vi "LSMcontroller_v59_PIzstage.vi"() -> ()   [LabVIEW 2015] (continued)
                                tunnel: w2761 -> [w2765 w2785]
                                tunnel: w2762 -> [_ w2791]
                                frame False {
                                w2769 = u16 0 items=["unsigned binary", "offset binary", "2's complement"] ("data format (offset binary)")
                                n482 = Initialize Array(sgl 0.0, w2765) -> (w2772:sgl[])
                                n483 = Replace Array Subset(array=w2772, new element=sgl 1.0, index=0) -> (w2770:sgl[])
                                n484 = Reciprocal(x=w2775) -> (1/x=w2776:sgl)
                                n485 = Bundle By Name("Y"=w2770, "dt"=w2776) -> (w2767:waveform(sgl))  [unwired: 1 in]
                                n486 = call-poly <vilib>:"Analog to Digital.vi"("data format (offset binary)"=w2769, "compress digital (T)"=TRUE, "full-scale range (pk-pk)"=1.0, "resolution (16 bit)"=1, "analog waveform"=w2767) -> ("digital waveform"=w2766:digitalwaveform)  [unwired: 3 in, 3 out]
                                }
                                frame True {
                                w2782 = u16 0 items=["unsigned binary", "offset binary", "2's complement"] ("data format (offset binary)")
                                n487 = To Double Precision Float(number=w2785) -> (double precision float=w2792:dbl)
                                n488 = Initialize Array(sgl 0.0, w2785) -> (w2787:sgl[])
                                n489 = Divide(x=w2791, y=w2792) -> (x/y=w2789:dbl)
                                n490 = Round Toward +Infinity(x=w2789) -> (ceil(x): smallest int >= x=w2790:dbl)
                                n491 = Replace Array Subset(array=w2787, new element=sgl 1.0, index=0) -> (w2784:sgl[])
                                n492 = for {
                                N: w2790 -> [_]
                                tunnel: w2784 -> [w2796]
                                tunnel: [w2796] -> w2793 mode=concatenating
                                }
                                n493 = Reciprocal(x=w2794) -> (1/x=w2795:sgl)
                                n494 = Bundle By Name("Y"=w2793, "dt"=w2795) -> (w2780:waveform(sgl))  [unwired: 1 in]
                                n495 = call-poly <vilib>:"Analog to Digital.vi"("data format (offset binary)"=w2782, "compress digital (T)"=TRUE, "full-scale range (pk-pk)"=1.0, "resolution (16 bit)"=1, "analog waveform"=w2780) -> ("digital waveform"=w2779:digitalwaveform)  [unwired: 3 in, 3 out]
                                }
                                }
                                n496 = Build Array (concatenate)(w2754, w2756) -> (w2752:digitalwaveform[])
                                n497 = call "waveformsDObuffer.vi"("DO wf in"=w2752, "command"="set") -> ()  [unwired: 1 out]
                                }
                                frame 2 {
                                n498 = call "waveformsDObuffer.vi"("command"="get") -> ("DO wf out"=w2800:digitalwaveform[])  [unwired: 1 in]
                                n499 = Delete From Array(array=w2800, length=1, index=w2803) -> (deleted portion=w2798:digitalwaveform[], array with subset deleted=w2797:digitalwaveform[])
                                n500 = call "waveformsDObuffer.vi"("DO wf in"=w2797, "command"="set") -> ()  [unwired: 1 out]
                                }
                                frame 3, Default {
                                }
                                frame 0 {
                                n501 = local read "Measurement"() -> (w2806:T4)
                                n502 = To Unsigned Long Integer(number=w2806) -> (unsigned 32bit integer=w2805:u32)
                                n503 = case shown="5..7" w2805 {
                                tunnel: w2807 -> [_ w2810]
                                tunnel: [_ w2809] -> w2804
                                frame 0..4, Default {
                                }
                                frame 5..7 {
                                n504 = call "2pparameters.vi"("command"="get") -> ("params out"=w2817:T11)  [unwired: 1 in]
                                n505 = Unbundle By Name(w2817) -> ("wavdet"=w2818:bool, "sAOxy"=w2820:i32, "refwfsize"=w2821:dbl, "srate Img"=w2819:sgl)
                                n506 = call "waveformsDObuffer.vi"("command"="get") -> ("DO wf out"=w2811:digitalwaveform[])  [unwired: 1 in]
                                n507 = Index Array(array=w2811, index=w2810) -> (element=w2812:digitalwaveform)
                                n508 = case shown="True" w2818 {
                                tunnel: [w2825 w2838] -> w2815
                                tunnel: w2819 -> [w2834 w2853]
                                tunnel: w2820 -> [w2824 w2844]
                                tunnel: w2821 -> [_ w2850]
                                frame False {
                                w2828 = u16 0 items=["unsigned binary", "offset binary", "2's complement"] ("data format (offset binary)")
                                n509 = Initialize Array(sgl 0.0, w2824) -> (w2831:sgl[])
                                n510 = Replace Array Subset(array=w2831, new element=sgl 1.0, index=0) -> (w2829:sgl[])
                                n511 = Reciprocal(x=w2834) -> (1/x=w2835:sgl)
                                n512 = Bundle By Name("Y"=w2829, "dt"=w2835) -> (w2826:waveform(sgl))  [unwired: 1 in]
                                n513 = call-poly <vilib>:"Analog to Digital.vi"("data format (offset binary)"=w2828, "compress digital (T)"=TRUE, "full-scale range (pk-pk)"=1.0, "resolution (16 bit)"=1, "analog waveform"=w2826) -> ("digital waveform"=w2825:digitalwaveform)  [unwired: 3 in, 3 out]
                                }
                                frame True {
                                w2841 = u16 0 items=["unsigned binary", "offset binary", "2's complement"] ("data format (offset binary)")
                                n514 = To Double Precision Float(number=w2844) -> (double precision float=w2851:dbl)
                                n515 = Initialize Array(sgl 0.0, w2844) -> (w2846:sgl[])
                                n516 = Divide(x=w2850, y=w2851) -> (x/y=w2848:dbl)
                                n517 = Round Toward +Infinity(x=w2848) -> (ceil(x): smallest int >= x=w2849:dbl)
                                n518 = Replace Array Subset(array=w2846, new element=sgl 1.0, index=0) -> (w2843:sgl[])
                                n519 = for {
                                N: w2849 -> [_]
                                tunnel: w2843 -> [w2855]
                                tunnel: [w2855] -> w2852 mode=concatenating
                                }
                                n520 = Reciprocal(x=w2853) -> (1/x=w2854:sgl)
                                n521 = Bundle By Name("Y"=w2852, "dt"=w2854) -> (w2839:waveform(sgl))  [unwired: 1 in]
                                n522 = call-poly <vilib>:"Analog to Digital.vi"("data format (offset binary)"=w2841, "compress digital (T)"=TRUE, "full-scale range (pk-pk)"=1.0, "resolution (16 bit)"=1, "analog waveform"=w2839) -> ("digital waveform"=w2838:digitalwaveform)  [unwired: 3 in, 3 out]
                                }
                                }
                                n523 = Build Array(w2812) -> (w2809:digitalwaveform[])
                                n524 = Replace Array Subset(array=w2811, new element=w2815, index=w2810) -> (w2808:digitalwaveform[])
                                n525 = call "waveformsDObuffer.vi"("DO wf in"=w2808, "command"="set") -> ()  [unwired: 1 out]
                                }
                                }
                                }
                                }
                              }
                              frame #10 {
                                n526 = local read "Meastab"() -> (w2870:enum32{"X-Y Image", "Linescan", "Timetrace"})
                                n527 = property on="refwf" class="Ring (strict)"() -> ("RingText.Text"=w2867:string)  [unwired: 2 in, 2 out]
                                n528 = case shown="\"Timetrace\"" w2870 {
                                tunnel: [w2872 w2873] -> w2871
                                frame "X-Y Image", Default {
                                n529 = local read "Sampling rate"() -> (w2872:dbl)
                                }
                                frame "Timetrace" {
                                n530 = local read "srateAODOtt"() -> (w2873:dbl)
                                }
                                }
                                n531 = call "waveformsAObuffer.vi"("command"="get") -> ("AO wf out"=w2858:waveform(dbl)[])  [unwired: 1 in]
                                n532 = local read "wavdet"() -> (w2868:bool)
                                n533 = call "waveformsDObuffer.vi"("command"="get") -> ("DO wf out"=w2862:digitalwaveform[])  [unwired: 1 in]
                                n534 = call "correctwaveformsizetemp.vi"("new sampling frequency (Hz)"=w2871, "start"=TRUE, "reference waveforms to"=w2867, "Analog waveforms in"=w2858, "stop"=FALSE, "Digital waveforms in"=w2862) -> ("analog wf out"=w2864:waveform(dbl)[], "Digital wf out"=w2866:digitalwaveform[], "measpoints"=w2869:i32)
                                n535 = call "GetNumCamFramesv2.vi"("Digital Waveform Graph"=w2866) -> ("Numeric"=w2865:i32)  [unwired: 10 in]
                                n536 = call "waveformsDObuffer.vi"("DO wf in"=w2866, "command"="set") -> ()  [unwired: 1 out]
                                n537 = call "waveformsAObuffer.vi"("AO wf in"=w2864, "command"="set") -> ()  [unwired: 1 out]
                                n538 = local write "Total Camera Frames"(w2865) -> ()
                                n539 = case shown="True" w2868 {
                                tunnel: w2869 -> [_ w2874]
                                frame False {
                                }
                                frame True {
                                n540 = local write "# of frames"(w2874) -> ()
                                }
                                }
                              }
                            }
                          }
                          frame #6 {
                            # "Disabled for conversion to 64 bit"
                            n541 = disable-structure shown="Disabled" {
                              frame Disabled {
                                n542 = local read "Measurement"() -> (w2879:T4)
                                n543 = case shown="\"Lifetime (scan)\"" w2879 {
                                frame "X-Y-t movie", Default {
                                }
                                frame "Lifetime (scan)" {
                                # "total acquisition time"
                                n544 = call "2pparameters.vi"("command"="get") -> ("params out"=w2885:T11)  [unwired: 1 in]
                                n545 = Unbundle By Name(w2885) -> ("measpoints"=w2906:i32, "avpp"=w2907:i32, "sAOxy"=w2886:i32, "srate Img"=w2908:sgl)
                                n546 = Multiply(x=w2906, y=w2907) -> (x*y=w2904:i32)
                                n547 = To Double Precision Float(number=w2886) -> (double precision float=w2891:dbl)
                                n548 = Divide(x=w2891, y=w2908) -> (x/y=w2893:dbl)
                                n549 = To Double Precision Float(number=w2904) -> (double precision float=w2889:dbl)
                                n550 = local read "min phot"() -> (w2900:u32)
                                n551 = local read "expected c/s"() -> (w2901:dbl)
                                n552 = Multiply(x=w2889, y=w2893) -> (x*y=w2887:dbl)
                                n553 = Multiply(x=w2887, y=1000.0) -> (x*y=w2892:dbl)
                                n554 = local read "Ch1 ZeroX"() -> (w2898:i32)
                                n555 = local read "truncate"() -> (w2899:u32)
                                n556 = To Long Integer(number=w2892) -> (32bit integer=w2902:i32)
                                n557 = To Long Integer(number=w2901) -> (32bit integer=w2903:i32)
                                n558 = local read "Number of Bins"() -> (w2894:u32)
                                n559 = local read "Ch1 Level"() -> (w2896:i32)
                                n560 = local read "Ch0 ZeroX"() -> (w2897:i32)
                                n561 = local write "Acquisition time"(w2902) -> ()
                                n562 = local read "Ch0 Level"() -> (w2895:i32)
                                n563 = call "lifetimeparameters.vi"("command"="get") -> ("Params out"=w2883:T20)  [unwired: 1 in]
                                n564 = Add(x=10, y=w2902) -> (x+y=w2890:i32)
                                n565 = Bundle By Name(cluster=w2883, "acq time"=w2890, "acq rate"=w2903, "# bins"=w2894, "Ch0 Level"=w2895, "Ch1 Level"=w2896, "Ch0 ZeroX"=w2897, "Ch1 ZeroX"=w2898, "min photons"=w2900, "truncate"=w2899) -> (w2882:T20)
                                n566 = local write "Acquisition rate"(w2903) -> ()
                                n567 = call "lifetimeparameters.vi"("Params in"=w2882, "command"="set") -> ()  [unwired: 1 out]
                                }
                                }
                                n568 = local read "min phot"() -> (w2877:u32)
                                n569 = Decrement(x=w2877) -> (x-1=w2878:u32)
                                n570 = To Double Precision Float(number=w2878) -> (double precision float=w2876:dbl)
                                n571 = property on="img_CH1" class="IntGraph (strict)"("ZScale.Minimum"=w2876) -> ()  [unwired: 2 in, 2 out]
                              }
                              frame Enabled {
                              }
                            }
                            n572 = local write "64bit disabled"(TRUE ("64bit disabled")) -> ()
                          }
                          frame #7 {
                            n573 = local read "Sampling rate"() -> (w2910:dbl)
                            n574 = call "calcdaqtime.vi"("sampling rate"=w2910) -> ("Calc. time per frame (ms)"=w2909:dbl)
                            n575 = local write "Calc. time per frame (ms)"(w2909) -> ()
                          }
                          frame #8 {
                            n576 = call "2pparameters.vi"("command"="get") -> ("params out"=w2921:T11)  [unwired: 1 in]
                            n577 = local read "Measurement"() -> (w2912:T4)
                            n578 = Unbundle By Name(w2921) -> ("bufferAI"=w2919:i32, "srate"=w2920:sgl)
                            n579 = To Double Precision Float(number=w2919) -> (double precision float=w2913:dbl)
                            n580 = To Double Precision Float(number=w2920) -> (double precision float=w2923:dbl)
                            n581 = case shown="\"X-Y-t movie\", Default" w2912 {
                              tunnel: [w2928 w2932] -> w2911
                              frame "X-Y-t movie", Default {
                                n582 = local read "wavdet"() -> (w2929:bool)
                                n583 = case shown="False" w2929 {
                                tunnel: [w2930 w2931] -> w2928
                                frame False {
                                w2930 = 10123 items=["Finite Samples"=10178, "Continuous Samples"=10123, "Hardware Timed Single Point"=12522] ("sample mode")
                                }
                                frame True {
                                w2931 = 10123 items=["Finite Samples"=10178, "Continuous Samples"=10123, "Hardware Timed Single Point"=12522] ("sample mode")
                                }
                                }
                              }
                              frame "X-Y-Z stack" {
                                w2932 = 10178 items=["Finite Samples"=10178, "Continuous Samples"=10123, "Hardware Timed Single Point"=12522] ("sample mode")
                              }
                            }
                            n584 = Divide(x=w2913, y=w2923) -> (x/y=w2927:dbl)
                            n585 = Multiply(x=w2927, y=2.0) -> (x*y=w2924:dbl)
                            n586 = Max & Min(x=w2924, y=10.0) -> (max(x,y)=w2914:dbl)  [unwired: 1 out]
                            n587 = call "2pparameters.vi"("command"="get") -> ("params out"=w2918:T11)  [unwired: 1 in]
                            n588 = Bundle By Name(cluster=w2918, "timeout"=w2914, "sample mode"=w2911) -> (w2915:T11)
                            n589 = call "2pparameters.vi"("Params in"=w2915, "command"="set") -> ()  [unwired: 1 out]
                          }
                          frame #9 {
                            n590 = local read "# of frames"() -> (w2933:i32)
                            n591 = call "timestamps.vi"("# of frames"=w2933, "command"="init") -> ()  [unwired: 2 in, 1 out]
                          }
                        }
                      }
                      frame #2 {
                        # "Disabled for conversion to 64 bit"
                        n592 = call "prepAO_img.vi"() -> ("Terminal Name with Device Prefix"=w2936:tag)
                        n593 = call "prepAI_img.vi"("triggersource"=w2936) -> ()  [unwired: 2 in]
                        n594 = call "prepCI_img.vi"("ArmStart.DigEdge.Src"=w2936) -> ()  [unwired: 1 in]
                        n595 = call "prepDO_img.vi"() -> ()  [unwired: 2 in]
                        n596 = disable-structure shown="Disabled" {
                          frame Disabled {
                            n597 = local read "Measurement"() -> (w2937:T4)
                            n598 = case shown="\"Lifetime (scan)\"" w2937 {
                              frame "X-Y-t movie", Default {
                              }
                              frame "Lifetime (scan)" {
                                n599 = stacked-sequence {
                                frame #0 {
                                n600 = call "PH-temp.vi"("String"="clear" ("command")) -> ()  [unwired: 2 in, 2 out]
                                n601 = call "PH-temp-raw.vi"("command"="empty") -> ()  [unwired: 1 in, 1 out]
                                }
                                frame #1 {
                                n602 = call "calib.vi"() -> ()  [unwired: 1 in]
                                }
                                frame #2 {
                                n603 = call "setup.vi"() -> ()  [unwired: 1 in]
                                }
                                }
                              }
                            }
                          }
                          frame Enabled {
                          }
                        }
                        n604 = local write "64bit disabled"(TRUE ("64bit disabled")) -> ()
                      }
                      frame #3 {
                        n605 = local read "save\ndata"() -> (w2940:bool)
                        n606 = case shown="True" w2940 {
                          tunnel: w2941 -> [_ w2945]
                          frame False {
                          }
                          frame True {
                            n607 = local read "filename prefix"() -> (w2943:string)
                            n608 = local read "data dir"() -> (w2944:path)
                            n609 = call "preparetiffs.vi"("filename prefix"=w2943, "data dir"=w2944, "timestamp"=w2945) -> ("full-filename"=w2942:string)  [unwired: 1 in]
                            n610 = local write "full-filename"(w2942) -> ()
                          }
                        }
                        n611 = call "preptempbuffers.vi"() -> ()  [unwired: 12 in]
                      }
                      frame #4 {
                        # "Disabled Thorlabs Zstage;\nneeds to be replaced by PI code"
                        n612 = local read "Measurement"() -> (w2946:T4)
                        n613 = case shown="\"X-Y-Z stack\"" w2946 {
                          frame "X-Y-t movie", Default {
                          }
                          frame "X-Y-Z stack" {
                            # "Move Z stage"
                            n614 = local read "Z-Start (um)"() -> (w2952:dbl)
                            n615 = local read "Z-end (um)"() -> (w2951:dbl)
                            n616 = local read "# of frames"() -> (w2953:i32)
                            n617 = call "calcZslice.vi"("current slice"=0, "# of Slices"=w2953, "Z-Start (um)"=w2952, "Z-end (um)"=w2951) -> ("zpos (V)"=w2948:dbl, "zpos (um)"=w2949:dbl)
                            n618 = call "moveZ_V2.vi"("Z"=w2948) -> ()
                            n619 = local write "Cal. Z"(w2949) -> ()
                          }
                        }
                        n620 = local write "Thorlabs Zstage disabled"(TRUE ("64bit disabled")) -> ()
                      }
                      frame #5 {
                        n621 = flat-sequence {
                          frame #0 {
                            n622 = call "2pparameters.vi"("command"="get") -> ("params out"=w2955:T11)  [unwired: 1 in]
                            n623 = Unbundle By Name(w2955) -> ("autoshutter"=w2956:bool)
                            n624 = case shown="True" w2956 {
                              frame False {
                              }
                              frame True {
                                n625 = call "shuttercontrol.vi"("command"="open") -> ()  [unwired: 1 in, 1 out]
                              }
                            }
                          }
                          frame #1 {
                            n626 = call "2pparameters.vi"("command"="get") -> ("params out"=w2960:T11)  [unwired: 1 in]
                            n627 = Tick Count (ms)() -> (millisecond timer value=w2959:u32)
                            n628 = Bundle By Name(cluster=w2960, "starttick"=w2959) -> (w2958:T11)
                            n629 = call "2pparameters.vi"("Params in"=w2958, "command"="set") -> ()  [unwired: 1 out]
                          }
                        }
                      }
                      frame #6 {
                        n630 = local read "Measurement"() -> (w2963:T4)
                        n631 = case shown="\"Lifetime (scan)\"" w2963 {
                          frame "X-Y-t movie" {
                            n632 = flat-sequence {
                              frame #0 {
                                n633 = call "runAI_img.vi"() -> ()  [unwired: 12 in]
                                n634 = call "runCI.vi"() -> ()  [unwired: 12 in]
                                n635 = call "runDO_img.vi"() -> ()  [unwired: 12 in]
                              }
                              frame #1 {
                                n636 = call "runAO_img.vi"() -> ()  [unwired: 12 in]
                              }
                            }
                          }
                          frame "Lifetime (scan)" {
                            # "Disabled for conversion to 64 bit"
                            n637 = disable-structure shown="Disabled" {
                              frame Disabled {
                                n638 = flat-sequence {
                                frame #0 {
                                n639 = call "runLT_img.vi"() -> ()  [unwired: 1 in]
                                n640 = call "runDO_img.vi"() -> ()  [unwired: 12 in]
                                }
                                frame #1 {
                                n641 = call "runAI_img.vi"() -> ()  [unwired: 12 in]
                                n642 = call "runCI.vi"() -> ()  [unwired: 12 in]
                                }
                                frame #2 {
                                n643 = call "runAO_img.vi"() -> ()  [unwired: 12 in]
                                }
                                }
                              }
                              frame Enabled {
                              }
                            }
                            n644 = local write "64bit disabled"(TRUE ("64bit disabled")) -> ()
                          }
                          frame "X-Y-Z stack", Default {
                          }
                        }
                      }
                      frame #7 {
                        # "Disabled for conversion to 64 bit"
                        n645 = while {
                          i -> [w2992]
                          stop <- w2989 stop-if-true
                          n646 = local read "Exit"() -> (w2997:bool)
                          n647 = local read "Stop"() -> (w2988:bool)
                          n648 = Or(x=w2988, y=w2997) -> (x .or. y?=w2993:bool)
                          n649 = case shown="False" w2993 {
                            tunnel: w2992 -> [w2998 _]
                            frame False {
                              n650 = stacked-sequence {
                                seq-local: [w3000 _ _ _ _ _ _] -> [_ _ _ _ _ _ w3116]
                                seq-local: [w2999 _ _ _ _ _ _] -> [_ _ _ _ _ _ w3115]
                                tunnel: w2998 -> [_ w3006 _ _ _ _ _]
                                frame #0 {
                                n651 = local read "Live"() -> (w3001:bool)
                                n652 = case shown="True" w3001 {
                                tunnel: [_ w3003] -> w3000
                                tunnel: [_ w3002] -> w2999
                                frame False {
                                }
                                frame True {
                                n653 = local read "Laserpower \n(%)"() -> (w3002:dbl)
                                n654 = local read "lpow"() -> (w3003:dbl)
                                }
                                }
                                n655 = call "preptempbuffers.vi"() -> ()  [unwired: 12 in]
                                }
                                frame #1 {
                                # "Move in Z if necessary"
                                # "Disabled Thorlabs Zstage;\nneeds to be replaced by PI code"
                                n656 = local read "Measurement"() -> (w3004:T4)
                                n657 = case shown="\"X-Y-Z stack\"" w3004 {
                                tunnel: w3006 -> [_ w3008]
                                frame "X-Y-t movie", Default {
                                }
                                frame "X-Y-Z stack" {
                                n658 = local read "Z-Start (um)"() -> (w3010:dbl)
                                n659 = local read "Z-end (um)"() -> (w3009:dbl)
                                n660 = local read "# of frames"() -> (w3011:i32)
                                n661 = call "calcZslice.vi"("current slice"=w3008, "# of Slices"=w3011, "Z-Start (um)"=w3010, "Z-end (um)"=w3009) -> ("zpos (um)"=w3007:dbl)  [unwired: 1 out]
                                n662 = local write "Cal. Z"(w3007) -> ()
                                }
                                }
                                n663 = local write "Thorlabs Zstage disabled"(TRUE ("64bit disabled")) -> ()
                                }
                                frame #2 {
                                # "main loop"
                                n664 = for {
                                N: "avpp" -> [_]
                                i -> [w3017]
                                n665 = local read "Stop"() -> (w3015:bool)
                                n666 = local read "Exit"() -> (w3014:bool)
                                n667 = Increment(x=w3017) -> (x+1=w3016:i32)
                                n668 = Or(x=w3015, y=w3014) -> (x .or. y?=w3013:bool)
                                n669 = case shown="False" w3013 {
                                tunnel: w3016 -> [w3018 _]
                                frame False {
                                n670 = stacked-sequence {
                                seq-local: [w3019 _ _ _ _ _ _] -> [_ _ _ w3032 w3044 w3052 _]
                                tunnel: w3018 -> [w3020 _ _ _ _ _ _]
                                frame #0 {
                                n671 = local read "Live"() -> (w3019:bool)
                                n672 = case shown="True" w3019 {
                                tunnel: w3020 -> [_ w3023]
                                frame False {
                                }
                                frame True {
                                # "collect timetag for current image\nplus curent average"
                                n673 = To Single Precision Float(number=w3023) -> (single precision float=w3021:sgl)
                                n674 = Tick Count (ms)() -> (millisecond timer value=w3022:u32)
                                n675 = local write "Tick for Frame"(w3022) -> ()
                                n676 = local write "Current Average"(w3021) -> ()
                                }
                                }
                                }
                                frame #1 {
                                n677 = local read "Measurement"() -> (w3024:T4)
                                n678 = case shown="\"X-Y-Z stack\"" w3024 {
                                frame "X-Y-t movie", Default {
                                }
                                frame "X-Y-Z stack" {
                                n679 = stacked-sequence {
                                frame #0 {
                                n680 = disable-structure shown="Disabled" {
                                frame Disabled {
                                n681 = call "2pparameters.vi"("command"="get") -> ("params out"=w3026:T11)  [unwired: 1 in]
                                n682 = Unbundle By Name(w3026) -> ("autoshutter"=w3027:bool)
                                n683 = case shown="True" w3027 {
                                frame False {
                                }
                                frame True {
                                n684 = call "shuttercontrol.vi"("command"="open") -> ()  [unwired: 1 in, 1 out]
                                }
                                }
                                }
                                frame Enabled {
                                }
                                }
                                }
                                frame #1 {
                                n685 = call "runAI_img.vi"() -> ()  [unwired: 12 in]
                                n686 = call "runCI.vi"() -> ()  [unwired: 12 in]
                                n687 = call "runDO_img.vi"() -> ()  [unwired: 12 in]
                                }
                                frame #2 {
                                n688 = call "runAO_img.vi"() -> ()  [unwired: 12 in]
                                }
                                }
                                }
                                }
                                }
                                frame #2 {
                                n689 = call "collectCI_img.vi"() -> ("Avg cts/s"=w3031:dbl, "recorded samples"=w3030:i32)  [unwired: 1 out]
                                n690 = call "collectAI_img.vi"() -> ("wrap"=w3029:i32)  [unwired: 3 in]
                                n691 = local write "scol"(w3030) -> ()
                                n692 = local write "wrap"(w3029) -> ()
                                n693 = local write "Avg Counts/s"(w3031) -> ()
                                }
                                frame #3 {
                                n694 = case shown="True" w3032 {
                                frame False {
                                }
                                frame True {
                                n695 = local read "Measurement"() -> (w3033:T4)
                                n696 = case shown="\"X-Y-t movie\", Default" w3033 {
                                frame "X-Y-t movie", Default {
                                n697 = local read "ROI Type"() -> (w3034:u16)
                                n698 = case shown="0" w3034 {
                                frame 0 {
                                # "display chosen channels"
                                n699 = local read "Current Average"() -> (w3043:sgl)
                                n700 = local read "image1list"() -> (w3039:u16)
                                n701 = local read "image2list"() -> (w3042:u16)
                                n702 = To Unsigned Word Integer(number=w3042) -> (unsigned 16bit integer=w3037:u16)
                                n703 = To Unsigned Word Integer(number=w3039) -> (unsigned 16bit integer=w3038:u16)
                                n704 = call "dattoimage.vi"("image2list"=w3037, "Current Average"=w3043, "image1list"=w3038) -> ("image 2 array out"=w3041:sgl[][], "image 1 array out"=w3040:sgl[][])
                                n705 = Transpose 2D Array(2D array=w3040) -> (transposed array=w3036:sgl[][])
                                n706 = Transpose 2D Array(2D array=w3041) -> (transposed array=w3035:sgl[][])
                                n707 = local write "img_CH1"(w3036) -> ()
                                n708 = local write "img_CH2"(w3035) -> ()
                                }
                                frame 1, Default {
                                }
                                }
                                }
                                frame "Lifetime (scan)" {
                                }
                                }
                                }
                                }
                                }
                                frame #4 {
                                n709 = case shown="True" w3044 {
                                frame False {
                                }
                                frame True {
                                # "set colormaps"
                                n710 = call "misc-global.vi"("command"="get") -> ("misc out"=w3048:cluster{"Colormaps":u32[][]})  [unwired: 1 in]
                                n711 = Unbundle By Name(w3048) -> ("Colormaps"=w3047:u32[][])
                                n712 = control-ref of="img_CH1"() -> (w3051:refnum<vi>)
                                n713 = control-ref of="img_CH2"() -> (w3050:refnum<vi>)
                                n714 = Index Array(array=w3047, index (row)="Colormap") -> (element=w3046:u32[])  [unwired: 1 in]
                                n715 = property class="IntGraph (strict)"(reference=w3051, "Color Table"=w3046) -> ()  [unwired: 1 in, 2 out]
                                n716 = property class="IntGraph (strict)"(reference=w3050, "Color Table"=w3046) -> ()  [unwired: 1 in, 2 out]
                                }
                                }
                                }
                                frame #5 {
                                n717 = case shown="True" w3052 {
                                frame False {
                                }
                                frame True {
                                # "crude estimate of time per frame\n(resolution is 1 ms), not so much for\nplotting purposes, more for debugging\ncollection and processing data"
                                n718 = local read "ypixels ref"() -> (w3057:i32)
                                n719 = local read "Tick for Frame"() -> (w3058:u32)
                                n720 = Tick Count (ms)() -> (millisecond timer value=w3059:u32)
                                n721 = To Double Precision Float(number=w3057) -> (double precision float=w3056:dbl)
                                n722 = Subtract(x=w3059, y=w3058) -> (x-y=w3054:u32)
                                n723 = To Double Precision Float(number=w3054) -> (double precision float=w3055:dbl)
                                n724 = local write "Meas. time per frame (ms)"(w3054) -> ()
                                n725 = Divide(x=w3055, y=w3056) -> (x/y=w3053:dbl)
                                n726 = local write "time per line (ms)"(w3053) -> ()
                                }
                                }
                                }
                                frame #6 {
                                n727 = local read "Measurement"() -> (w3060:T4)
                                n728 = case shown="\"X-Y-Z stack\"" w3060 {
                                frame "X-Y-t movie", Default {
                                }
                                frame "X-Y-Z stack" {
                                n729 = call "2pparameters.vi"("command"="get") -> ("params out"=w3062:T11)  [unwired: 1 in]
                                n730 = Unbundle By Name(w3062) -> ("autoshutter"=w3063:bool)
                                n731 = call "stopCI_img.vi"() -> ()  [unwired: 12 in]
                                n732 = call "stopAI_img.vi"() -> ()  [unwired: 12 in]
                                n733 = case shown="True" w3063 {
                                frame False {
                                }
                                frame True {
                                n734 = call "shuttercontrol.vi"("command"="close") -> ()  [unwired: 1 in, 1 out]
                                }
                                }
                                n735 = Wait (ms)(milliseconds to wait=u32 100) -> ()  [unwired: 1 out]
                                n736 = call "stopAO_img.vi"() -> ()  [unwired: 12 in]
                                n737 = call "stopDO_img.vi"() -> ()  [unwired: 12 in]
                                }
                                }
                                }
                                }
                                }
                                frame True {
                                }
                                }
                                }
                                }
                                frame #3 {
                                n738 = local read "Measurement"() -> (w3066:T4)
                                n739 = case shown="\"Lifetime (scan)\"" w3066 {
                                frame "X-Y-t movie", Default {
                                }
                                frame "Lifetime (scan)" {
                                w3069 = u16 2 items=["Stream to disk", "Post process", "real time process"] ("Ring")
                                n740 = local read "T3R Data processing"() -> (w3070:u16)
                                n741 = Equal?(x=w3070, y=w3069) -> (x = y?=w3068:bool)
                                n742 = case shown="True" w3068 {
                                frame False {
                                }
                                frame True {
                                n743 = disable-structure shown="Disabled" {
                                frame Disabled {
                                n744 = local read "lineshift"() -> (w3073:i32)
                                n745 = call "wrapcutlifetime.vi"("lineshift"=w3073) -> ("pt3img"=w3075:u16[][], "lifetimes"=w3074:sgl[][], "okay"=w3071:bool, "# of frames"=w3072:i32)
                                n746 = case shown="True" w3071 {
                                tunnel: w3075 -> [_ w3085]
                                tunnel: w3074 -> [_ w3083]
                                tunnel: w3072 -> [_ w3079]
                                frame False {
                                }
                                frame True {
                                # "lifetime"
                                # "intensity"
                                n747 = Transpose 2D Array(2D array=w3085) -> (transposed array=w3077:u16[][])
                                n748 = Transpose 2D Array(2D array=w3083) -> (transposed array=w3084:sgl[][])
                                n749 = local write "frames recorded"(w3079) -> ()
                                n750 = local read "counts"() -> (w3078:i32)
                                n751 = Array Max & Min(array=w3077) -> (max value=w3082:u16)  [unwired: 3 out]
                                n752 = To Single Precision Float(number=w3077) -> (single precision float=w3076:sgl[][])
                                n753 = local write "img_CH2"(w3084) -> ()
                                n754 = local write "img_CH1"(w3076) -> ()
                                n755 = Quotient & Remainder(x=w3078, y=w3079) -> (floor(x/y)=→"photons/frame":i32)  [unwired: 1 out]
                                n756 = To Double Precision Float(number=w3082) -> (double precision float=w3081:dbl)
                                n757 = property on="img_CH1" class="IntGraph (strict)"("ZScale.Maximum"=w3081) -> ()  [unwired: 2 in, 2 out]
                                }
                                }
                                }
                                frame Enabled {
                                }
                                }
                                }
                                }
                                }
                                }
                                n758 = local read "save\ndata"() -> (w3067:bool)
                                n759 = case shown="True" w3067 {
                                frame False {
                                }
                                frame True {
                                n760 = local read "Current Average"() -> (w3086:sgl)
                                n761 = call "savetiffs.vi"("current average"=w3086) -> ()
                                }
                                }
                                }
                                frame #4 {
                                n762 = local read "save\ndata"() -> (w3087:bool)
                                n763 = case shown="True" w3087 {
                                frame False {
                                }
                                frame True {
                                n764 = local read "points recorded"() -> (w3089:i32)
                                n765 = call "timestamps.vi"("points recorded"=w3089, "command"="add") -> ()  [unwired: 2 in, 1 out]
                                }
                                }
                                }
                                frame #5 {
                                n766 = local read "Live"() -> (w3090:bool)
                                n767 = case shown="True" w3090 {
                                frame False {
                                }
                                frame True {
                                n768 = local read "downright"() -> (w3095:bool)
                                n769 = local read "downleft"() -> (w3097:bool)
                                n770 = local read "upright"() -> (w3093:bool)
                                n771 = local read "upleft"() -> (w3091:bool)
                                n772 = local read "down"() -> (w3096:bool)
                                n773 = local read "right"() -> (w3094:bool)
                                n774 = local read "left"() -> (w3098:bool)
                                n775 = local read "up"() -> (w3092:bool)
                                n776 = Compound Arithmetic op=OR(w3091, w3092, w3093, w3094, w3095, w3096, w3097, w3098) -> (w3099:bool)
                                n777 = case shown="True" w3099 {
                                frame False {
                                }
                                frame True {
                                n778 = stacked-sequence {
                                frame #0 {
                                n779 = local read "downright"() -> (w3101:bool)
                                n780 = local read "downleft"() -> (w3103:bool)
                                n781 = local read "BigSmall"() -> (w3100:bool)
                                n782 = local read "upright"() -> (w3105:bool)
                                n783 = local read "upleft"() -> (w3108:bool)
                                n784 = local read "down"() -> (w3104:bool)
                                n785 = local read "right"() -> (w3106:bool)
                                n786 = local read "left"() -> (w3102:bool)
                                n787 = local read "up"() -> (w3107:bool)
                                n788 = call "movestageparams.vi"("command"="get") -> ("Params out"=w3111:T21)  [unwired: 1 in]
                                n789 = Bundle By Name(cluster=w3111, "upleft"=w3108, "up"=w3107, "upright"=w3105, "right"=w3106, "downright"=w3101, "down"=w3104, "downleft"=w3103, "left"=w3102, "Bigsmall"=w3100) -> (w3112:T21)
                                n790 = call "movestageparams.vi"("Params in"=w3112, "command"="set") -> ()  [unwired: 1 out]
                                }
                                frame #1 {
                                n791 = call "movestage.vi"() -> ()  [unwired: 12 in]
                                }
                                frame #2 {
                                w3113 = FALSE ("OK Button")
                                w3114 = FALSE ("OK Button")
                                n792 = property on="down" class="Bool (strict)"("Value"=w3114) -> ()  [unwired: 2 in, 2 out]
                                n793 = property on="up" class="Bool (strict)"("Value"=w3114) -> ()  [unwired: 2 in, 2 out]
                                n794 = property on="right" class="Bool (strict)"("Value"=w3114) -> ()  [unwired: 2 in, 2 out]
                                n795 = property on="left" class="Bool (strict)"("Value"=w3114) -> ()  [unwired: 2 in, 2 out]
                                n796 = property on="upright" class="Bool (strict)"("Value"=w3113) -> ()  [unwired: 2 in, 2 out]
                                n797 = property on="downleft" class="Bool (strict)"("Value"=w3113) -> ()  [unwired: 2 in, 2 out]
                                n798 = property on="downright" class="Bool (strict)"("Value"=w3113) -> ()  [unwired: 2 in, 2 out]
                                n799 = property on="upleft" class="Bool (strict)"("Value"=w3113) -> ()  [unwired: 2 in, 2 out]
                                }
                                }
                                }
                                }
                                }
                                }
                                }
                                frame #6 {
                                n800 = local read "Live"() -> (w3117:bool)
                                n801 = case shown="True" w3117 {
                                tunnel: w3116 -> [_ w3124]
                                tunnel: w3115 -> [_ w3123]
                                frame False {
                                }
                                frame True {
                                n802 = local read "Laserpower \n(%)"() -> (w3119:dbl)
                                n803 = local read "lpow"() -> (w3118:dbl)
                                n804 = Not Equal?(x=w3118, y=w3124) -> (x != y?=w3120:bool)
                                n805 = Not Equal?(x=w3119, y=w3123) -> (x != y?=w3121:bool)
                                n806 = Or(x=w3121, y=w3120) -> (x .or. y?=w3122:bool)
                                n807 = case shown="True" w3122 {
                                tunnel: w3121 -> [_ w3128]
                                tunnel: w3120 -> [_ w3127]
                                tunnel: w3119 -> [_ w3126]
                                tunnel: w3118 -> [_ w3125]
                                frame False {
                                }
                                frame True {
                                n808 = case shown="True" w3128 {
                                tunnel: w3126 -> [_ w3131]
                                frame False {
                                }
                                frame True {
                                n809 = local read "wavelength(nm)"() -> (w3132:dbl)
                                n810 = call "setpockelscellT.vi"("wavelength(nm)"=w3132, "transmission"=w3131) -> ()  [unwired: 1 in]
                                n811 = property on="lpow" class="DigNum (strict)"("Value"=w3131) -> ()  [unwired: 2 in, 2 out]
                                }
                                }
                                n812 = case shown="True" w3127 {
                                tunnel: w3125 -> [_ w3129]
                                frame False {
                                }
                                frame True {
                                n813 = local read "wavelength(nm)"() -> (w3130:dbl)
                                n814 = call "setpockelscellT.vi"("wavelength(nm)"=w3130, "transmission"=w3129) -> ()  [unwired: 1 in]
                                n815 = property on="Laserpower \n(%)" class="Slide (strict)"("Value"=w3129) -> ()  [unwired: 2 in, 2 out]
                                }
                                }
                                }
                                }
                                }
                                }
                                }
                              }
                            }
                            frame True {
                            }
                          }
                          n816 = Increment(x=w2992) -> (x+1=w2991:i32)
                          "points recorded" <- w2991
                          n817 = call "stopcond.vi"("prec"=w2991) -> ("stop"=w2990:bool)
                          n818 = local read "Stop"() -> (w2996:bool)
                          n819 = local read "Exit"() -> (w2995:bool)
                          n820 = Or(x=w2996, y=w2995) -> (x .or. y?=w2994:bool)
                          n821 = Or(x=w2990, y=w2994) -> (x .or. y?=w2989:bool)
                        }
                        n822 = disable-structure shown="Disabled" {
                          disable-tunnel: w2966 -> [w2972 _]
                          frame Disabled {
                            w2969 = u16 0 items=["Stream to disk", "Post process", "real time process"] ("Ring")
                            n823 = local read "T3R Data processing"() -> (w2968:u16)
                            n824 = Equal?(x=w2968, y=w2969) -> (x = y?=w2967:bool)
                            n825 = local read "save\ndata"() -> (w2971:bool)
                            n826 = local read "Measurement"() -> (w2973:T4)
                            n827 = And(x=w2971, y=w2967) -> (x .and. y?=w2970:bool)
                            n828 = case shown="\"Lifetime (scan)\"" w2973 {
                              tunnel: w2972 -> [_ w2977]
                              tunnel: w2970 -> [_ w2976]
                              frame "X-Y-t movie", Default {
                              }
                              frame "Lifetime (scan)" {
                                n829 = case shown="True" w2976 {
                                selector: w2976 -> [w2978 w2983]
                                tunnel: w2977 -> [_ w2981]
                                tunnel: [path "" ("appended path") w2984] -> w2975
                                tunnel: [w2978 w2983] -> w2974
                                frame False {
                                }
                                frame True {
                                n830 = local read "filename prefix"() -> (w2982:string)
                                n831 = local read "data dir"() -> (w2985:path)
                                n832 = call "generatedatafilename.vi"("timestamp"=w2981, "filename prefix in"=w2982) -> ("full-filename"=w2980:string)
                                n833 = Concatenate Strings(w2980, ".lvpt3img" ("string")) -> (w2987:string)
                                n834 = Build Path(base path=w2985, name or relative path=w2987) -> (appended path=w2984:path)
                                }
                                }
                                n835 = call "collectLT_img_v2.vi"("stream?"=w2974, "data file"=w2975) -> ()  [unwired: 2 out]
                              }
                            }
                          }
                          frame Enabled {
                          }
                        }
                        n836 = local write "64bit disabled"(TRUE ("64bit disabled")) -> ()
                      }
                      frame #8 {
                        # "Disabled for conversion to 64 bit"
                        n837 = local read "Measurement"() -> (w3135:T4)
                        n838 = case shown="\"Lifetime (scan)\"" w3135 {
                          tunnel: w3134 -> [_ _ w3136]
                          frame "X-Y-t movie", Default {
                          }
                          frame "X-Y-Z stack" {
                            n839 = call "eraseDO_img.vi"() -> ()  [unwired: 12 in]
                            n840 = call "eraseAO_img.vi"() -> ()  [unwired: 12 in]
                            n841 = call "eraseCI_img.vi"() -> ()  [unwired: 12 in]
                            n842 = call "eraseAI_img.vi"() -> ()  [unwired: 12 in]
                          }
                          frame "Lifetime (scan)" {
                            n843 = disable-structure shown="Disabled" {
                              disable-tunnel: w3136 -> [w3137 _]
                              frame Disabled {
                                n844 = stacked-sequence {
                                tunnel: w3137 -> [_ _ w3151 _ _]
                                frame #0 {
                                n845 = disable-structure shown="Disabled" {
                                frame Disabled {
                                n846 = call "stoperaseCI.vi"() -> ()  [unwired: 12 in]
                                n847 = call "stoperaseDO_img.vi"() -> ()  [unwired: 12 in]
                                n848 = call "stoperaseAO_img.vi"() -> ()  [unwired: 12 in]
                                n849 = call "stoperaseAI_img.vi"() -> ()  [unwired: 12 in]
                                }
                                frame Enabled {
                                }
                                }
                                }
                                frame #1 {
                                n850 = disable-structure shown="Disabled" {
                                frame Disabled {
                                n851 = local read "Acquisition time"() -> (w3141:i32)
                                n852 = call "collect_allLT_img.vi"() -> ("counts"=w3143:i32)  [unwired: 1 out]
                                n853 = local read "counts"() -> (w3144:i32)
                                n854 = Add(x=w3144, y=w3143) -> (x+y=w3142:i32)
                                "counts" <- w3142
                                n855 = Divide(x=w3142, y=w3141) -> (x/y=w3140:dbl)
                                n856 = Multiply(x=1000.0, y=w3140) -> (x*y=w3139:dbl)
                                n857 = local write "Avg Counts/s"(w3139) -> ()
                                }
                                frame Enabled {
                                }
                                }
                                }
                                frame #2 {
                                w3147 = u16 0 items=["Stream to disk", "Post process", "real time process"] ("Ring")
                                n858 = local read "T3R Data processing"() -> (w3146:u16)
                                n859 = local read "save\ndata"() -> (w3149:bool)
                                n860 = Equal?(x=w3146, y=w3147) -> (x = y?=w3145:bool)
                                n861 = Not(x=w3145) -> (.not. x?=w3150:bool)
                                n862 = And(x=w3149, y=w3150) -> (x .and. y?=w3148:bool)
                                n863 = case shown="True" w3148 {
                                tunnel: w3151 -> [_ w3153]
                                frame False {
                                }
                                frame True {
                                n864 = local read "filename prefix"() -> (w3154:string)
                                n865 = local read "data dir"() -> (w3159:path)
                                n866 = call "2pparameters.vi"("command"="get") -> ("params out"=w3174:T11)  [unwired: 1 in]
                                n867 = call "generatedatafilename.vi"("timestamp"=w3153, "filename prefix in"=w3154) -> ("full-filename"=w3152:string)
                                n868 = Unbundle By Name(w3174) -> ("srate"=w3172:sgl, "sAOxy"=w3171:i32, "Xpixels Img"=w3169:i32, "Ypixels Img"=w3167:i32)
                                n869 = Concatenate Strings(w3152, ".lvpt3img" ("string")) -> (w3157:string)
                                n870 = Build Path(base path=w3159, name or relative path=w3157) -> (appended path=w3156:path)
                                n871 = To Unsigned Long Integer(number=w3172) -> (unsigned 32bit integer=w3173:u32)
                                n872 = To Unsigned Long Integer(number=w3171) -> (unsigned 32bit integer=w3170:u32)
                                n873 = To Unsigned Long Integer(number=w3169) -> (unsigned 32bit integer=w3168:u32)
                                n874 = To Unsigned Long Integer(number=w3167) -> (unsigned 32bit integer=w3166:u32)
                                n875 = call "PH-temp-raw.vi"("command"="get") -> ("array out"=w3165:u32[])  [unwired: 1 in]
                                n876 = Build Array (concatenate)(w3173, w3170, w3168, w3166, w3165) -> (w3164:u32[])
                                n877 = Open/Create/Replace File(file path (use dialog)=w3156, operation (0:open)=T8."replace or create") -> (refnum out=w3163:refnum<file>, error out=w3162:errorcluster)  [unwired: 4 in, 1 out]
                                n878 = Write to Binary File(file (use dialog)=w3163, data=w3164, error in=w3162, 5:FALSE ("prepend array or string size? (T)")) -> (refnum out=w3160:refnum<file>, error out=w3161:errorcluster)  [unwired: 2 in, 1 out]
                                n879 = Close File(refnum=w3160, error in=w3161) -> ()  [unwired: 2 out]
                                }
                                }
                                n880 = call "stoperaseLT_img.vi"() -> ()  [unwired: 1 in]
                                }
                                frame #3 {
                                w3180 = u16 1 items=["Stream to disk", "Post process", "real time process"] ("Ring")
                                n881 = local read "T3R Data processing"() -> (w3179:u16)
                                n882 = Equal?(x=w3179, y=w3180) -> (x = y?=w3178:bool)
                                n883 = case shown="True" w3178 {
                                frame False {
                                }
                                frame True {
                                # "intensity"
                                # "lifetime"
                                # "intensity"
                                n884 = property on="img_CH1" class="IntGraph (strict)"() -> ("Value"=w3193:sgl[][])  [unwired: 2 in, 2 out]
                                n885 = Array Max & Min(array=w3193) -> (max value=w3194:sgl)  [unwired: 3 out]
                                n886 = local read "lineshift"() -> (w3181:i32)
                                n887 = local read "min phot"() -> (w3195:u32)
                                n888 = To Unsigned Long Integer(number=w3194) -> (unsigned 32bit integer=w3197:u32)
                                n889 = local read "counts"() -> (w3183:i32)
                                n890 = call "wrapcutlifetime.vi"("lineshift"=w3181) -> ("pt3img"=w3192:u16[][], "lifetimes"=w3190:sgl[][], "okay"=w3185:bool, "# of frames"=w3182:i32)
                                "frames recorded" <- w3182
                                n891 = Greater?(x=w3195, y=w3197) -> (0:w3196:bool)
                                n892 = Quotient & Remainder(x=w3183, y=w3182) -> (floor(x/y)=w3184:i32)  [unwired: 1 out]
                                n893 = Transpose 2D Array(2D array=w3192) -> (transposed array=w3186:u16[][])
                                n894 = Transpose 2D Array(2D array=w3190) -> (transposed array=w3191:sgl[][])
                                n895 = And(x=w3196, y=w3185) -> (x .and. y?=w3198:bool)
                                n896 = local write "img_CH2"(w3191) -> ()
                                n897 = local write "photons/frame"(w3184) -> ()
                                n898 = Array Max & Min(array=w3186) -> (max value=w3187:u16)  [unwired: 3 out]
                                n899 = To Single Precision Float(number=w3186) -> (single precision float=w3189:sgl[][])
                                n900 = case shown="True" w3198 {
                                tunnel: w3197 -> [_ w3202]
                                frame False {
                                }
                                frame True {
                                n901 = Quotient & Remainder(x=w3202, y=u32 2 ("min phot")) -> (floor(x/y)=w3201:u32)  [unwired: 1 out]
                                n902 = Max & Min(x=w3201, y=u32 5) -> (max(x,y)=w3200:u32)  [unwired: 1 out]
                                n903 = local write "min phot"(w3200) -> ()
                                }
                                }
                                n904 = To Double Precision Float(number=w3187) -> (double precision float=w3188:dbl)
                                n905 = local write "img_CH1"(w3189) -> ()
                                n906 = property on="img_CH1" class="IntGraph (strict)"("ZScale.Maximum"=w3188) -> ()  [unwired: 2 in, 2 out]
                                }
                                }
                                }
                                frame #4 {
                                w3206 = u16 1 items=["Stream to disk", "Post process", "real time process"] ("Ring")
                                n907 = local read "T3R Data processing"() -> (w3205:u16)
                                n908 = Equal?(x=w3205, y=w3206) -> (x = y?=w3204:bool)
                                n909 = case shown="False" w3204 {
                                frame False {
                                # "intensity"
                                n910 = local read "Current Average"() -> (w3211:sgl)
                                n911 = local read "image2list"() -> (w3207:u16)
                                n912 = local read "image1list"() -> (w3208:u16)
                                n913 = call "dattoimage.vi"("image2list"=w3207, "Current Average"=w3211, "image1list"=w3208) -> ("image 1 array out"=w3210:sgl[][])  [unwired: 1 out]
                                n914 = Transpose 2D Array(2D array=w3210) -> (transposed array=w3209:sgl[][])
                                n915 = local write "img_CH2"(w3209) -> ()
                                }
                                frame True {
                                }
                                }
                                }
                                }
                              }
                              frame Enabled {
                              }
                            }
                          }
                        }
